vi "GetParam.vi"(8 "error in (no error)":errorcluster caption="entrée d'erreur (pas d'erreur)", 11 "Circles.lvclass":refnum<class "Circles.lvclass">) -> (0 "error out":errorcluster caption="sortie d'erreur", 2 "make_circles":T1={"n_samples"="100", "shuffle"=TRUE, "noise"=-1.0, "random_state"=-1, "factor"=0.8, "Returns"="X"} {"factor" min=0.0 max=1.0; "noise" min=-1.0; "random_state" min=-1}, 3 "Circles.lvclass":refnum<class "Circles.lvclass">)   [LabVIEW 2020, in "Circles.lvclass"]
doc: "Get Parameters"
uses:
  Circles.lvclass
  Circles.lvclass/Circles.ctl
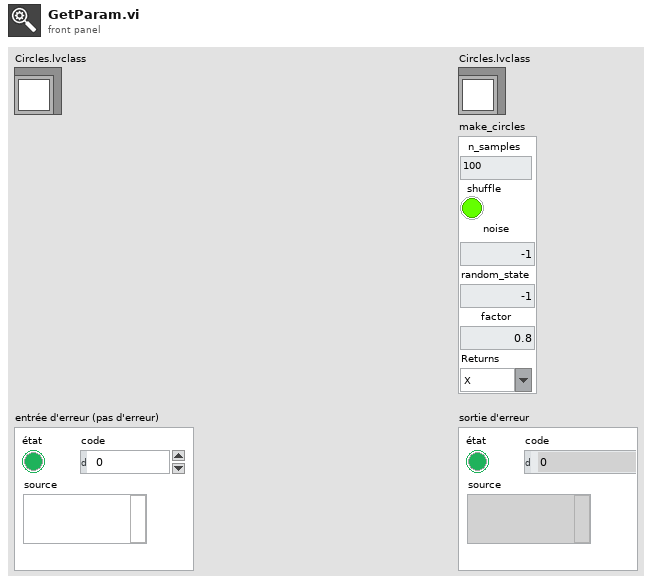
[diagram p1: front panel]
types:
  T1 = cluster{"n_samples":string, "shuffle":bool, "noise":dbl, "random_state":i32, "factor":dbl, "Returns":string}
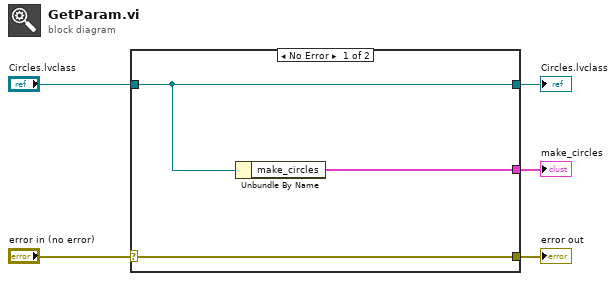
[diagram p0: block diagram]
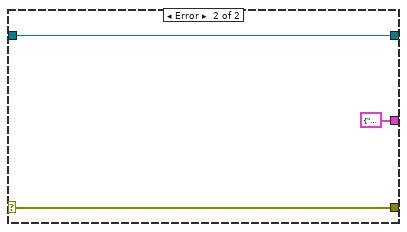
[diagram p2: hidden frame]
diagram:
  n1 = case shown="No Error" "error in (no error)" {
    selector: "error in (no error)" -> [w8 w10]
    tunnel: [w8 w10] -> w4
    tunnel: [w7 w11] -> w2
    tunnel: "Circles.lvclass" -> [w7 w11]
    tunnel: [w6 T1 {"n_samples"="", "shuffle"=FALSE, "noise"=0.0, "random_state"=0, "factor"=0.0, "Returns"=""} ("make_circles")] -> w1
    frame No Error {
      n2 = Unbundle By Name(w7) -> ("make_circles"=w6:T1)
    }
    frame Error {
    }
  }
  "error out" <- w4
  "Circles.lvclass" <- w2
  "make_circles" <- w1
